vi "GetType.vi"(8 "error in (no error)":errorcluster, 11 "Configure Operation Mode Msg in":refnum<class "Configure Operation Mode Msg.lvclass">) -> (0 "error out":errorcluster, 2 "Data Sample":variant, 3 "Configure Operation Mode Msg out":refnum<class "Configure Operation Mode Msg.lvclass">)   [LabVIEW 2014, in "CS++Fgen.lvlib" / "Configure Operation Mode Msg.lvclass"]
doc: "This VI delivers a sample of the data type format the message expects."
uses:
  Configure Operation Mode Msg.lvclass
  Configure Operation Mode Msg.lvclass/Configure Operation Mode Msg.ctl
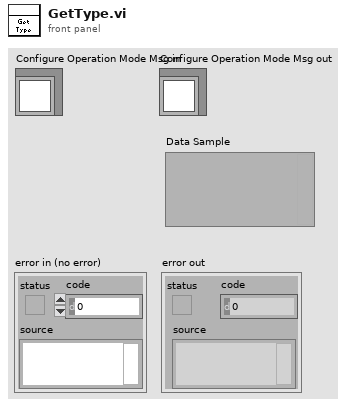
[diagram p1: front panel]
types:
  T1 = cluster{"channel name (\"CHANNEL1\")":string, "operation mode (Continuous)":i32}
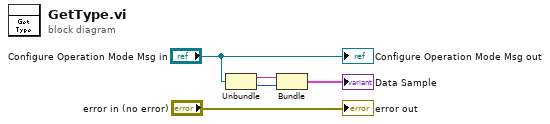
[diagram p0: block diagram]
diagram:
  n1 = Unbundle("Configure Operation Mode Msg in") -> (w3:string, w2:i32)
  n2 = Bundle("channel name (\"CHANNEL1\")"=w3, "operation mode (Continuous)"=w2) -> (→"Data Sample":T1)  [unwired: 1 in]
  "error out" <- "error in (no error)"
  "Configure Operation Mode Msg out" <- "Configure Operation Mode Msg in"
